vi "更新update.vi"() -> ()   [LabVIEW 2016, in "自动更新.lvlib"]
panel:
  out "waittime":u8
  out "下载的文件名":string
  out "更新进度":u8(slide) scale=0.0..100.0
  # "更新update，请稍后！"
  # "s"
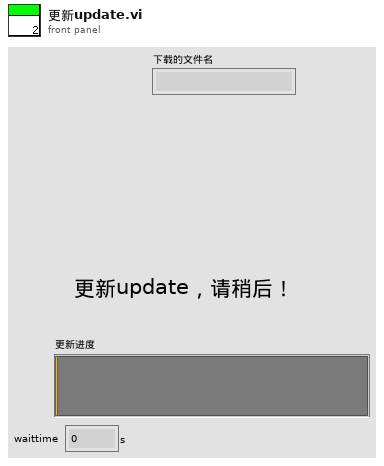
[diagram p1: front panel]
types:
  T1 = enum16{"get version information", "get success", "contact", "over"}
  T2 = cluster{"网络灯":bool, "接收中":bool, "已接收百分比":u8, "接收成功次数":dbl, "当前步骤":enum16{"init", "receivehead", "receivecontent", "receivesuccess", "over"}, "文件名":string, "error out":errorcluster}
  T3 = enum32{"Bad", "Idle", "Run top level", "Running"}
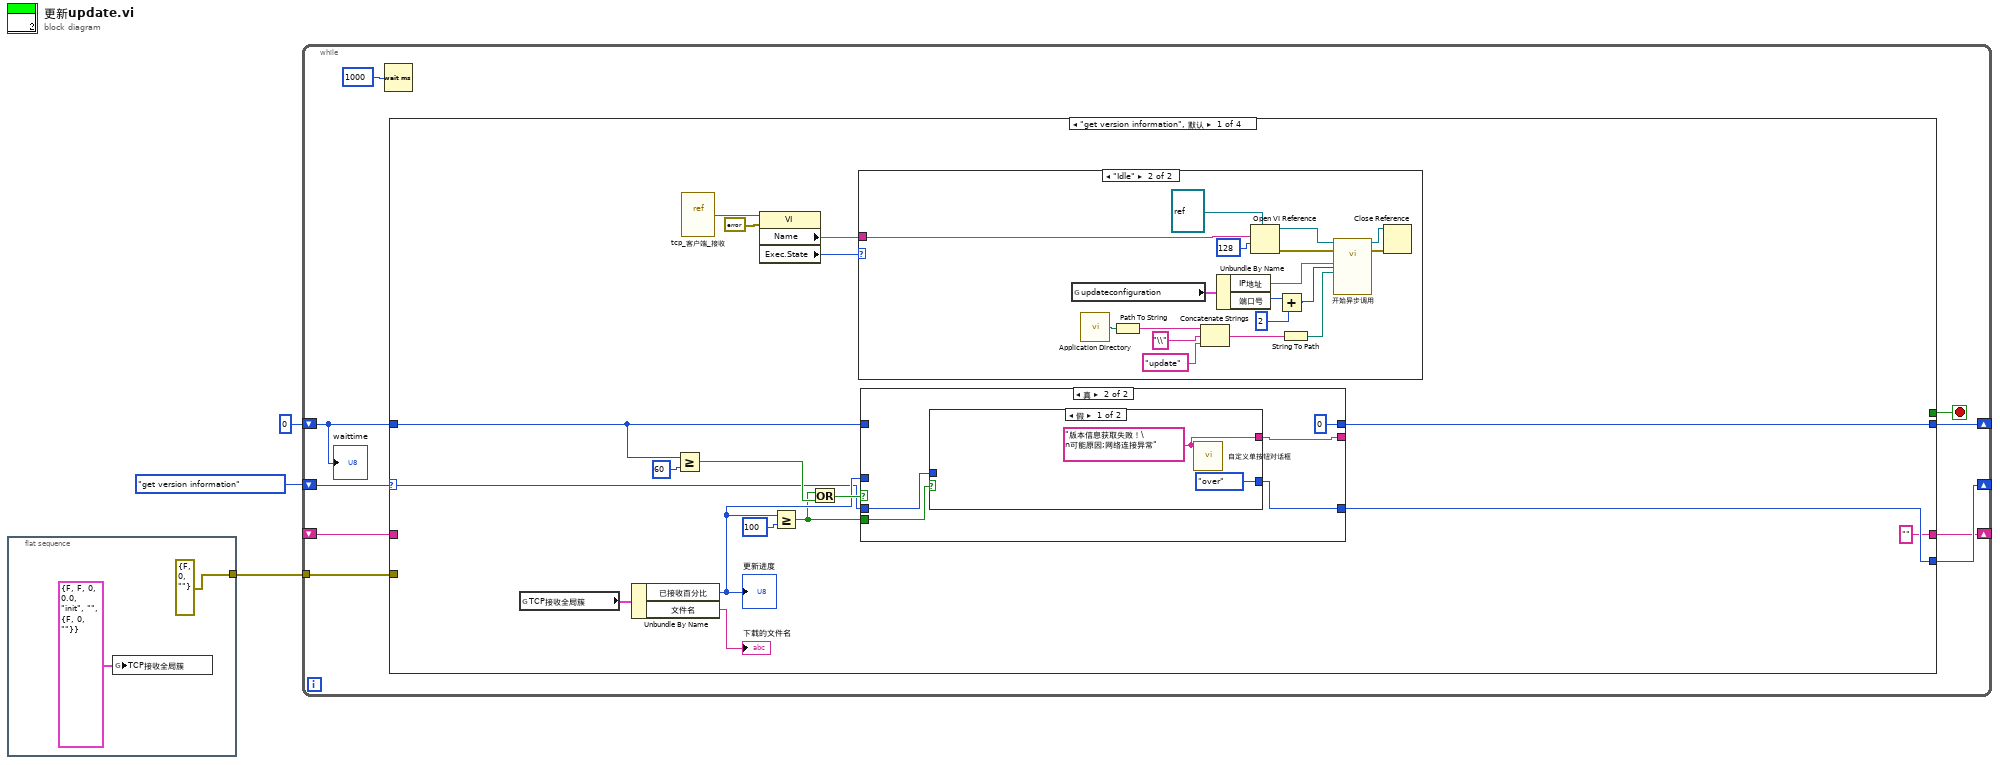
[diagram p0: block diagram]
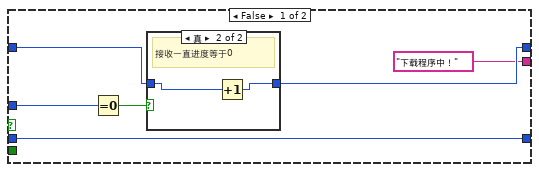
[diagram p2: hidden frame]
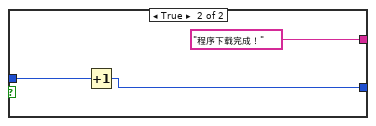
[diagram p4: hidden frame]
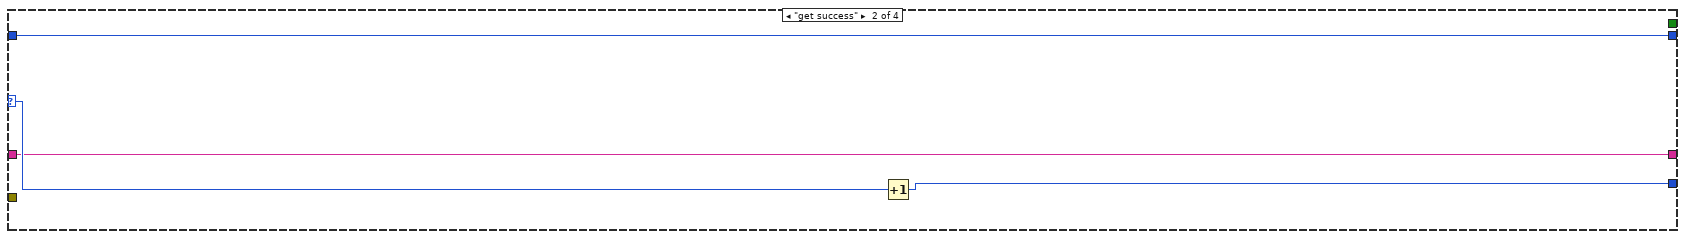
[diagram p6: hidden frame]
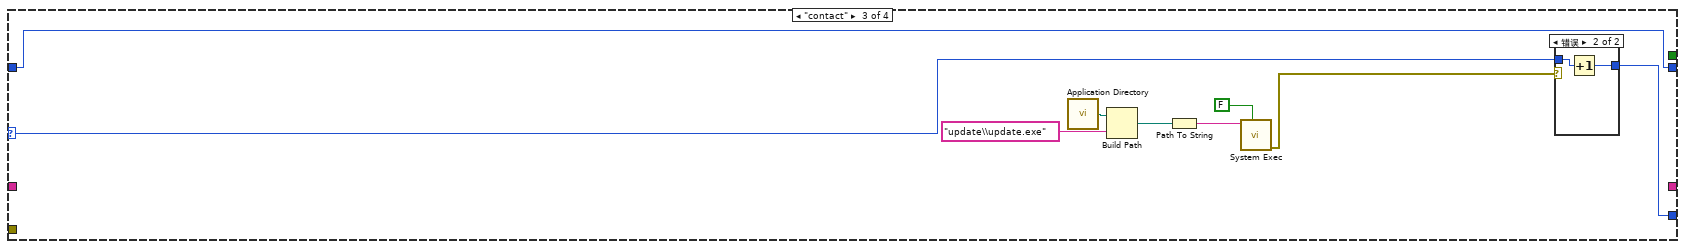
[diagram p7: hidden frame]
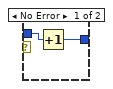
[diagram p8: hidden frame]
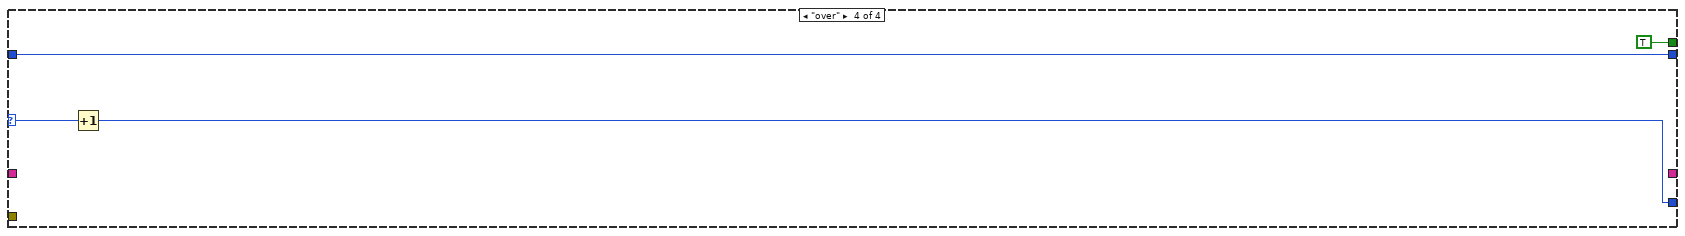
[diagram p9: hidden frame]
diagram:
  n1 = flat-sequence {
    tunnel: [errorcluster {"status"=FALSE, "code"=0, "source"=""} ("错误常量")] -> w1
    frame #0 {
      n2 = global write "全局变量1.vi" "TCP接收全局簇"(T2 {"网络灯"=FALSE, "接收中"=FALSE, "已接收百分比"=0, "接收成功次数"=0.0, "当前步骤"=enum."init", "文件名"="", "error out"={"status"=FALSE, "code"=0, "source"=""}} ("TCP接收全局簇")) -> ()
    }
  }
  n3 = while {
    shift-right: [w10] -> _
    shift-left: T1."get version information" -> [w13]
    shift-right: [w11] -> _
    shift-left: u8 0 ("y") -> [w12]
    tunnel: w1 -> [w9]
    shift-right: [w8] -> _
    shift-left: _ -> [w7]
    stop <- w6 stop-if-true
    n4 = Wait (ms)(milliseconds to wait=u32 1000 ("等待时间（毫秒）")) -> ()  [unwired: 1 out]
    n5 = case shown="\"get version information\", 默认" w13 {
      selector: w13 -> [w17 w71 w74 w87]
      tunnel: w12 -> [w19 w72 w80 w88]
      tunnel: [w18 w72 w80 w88] -> w11
      tunnel: [w16 w70 w81 w86] -> w10
      tunnel: w9 -> [_ _ _ _]
      tunnel: ["" w69 _ _] -> w8
      tunnel: w7 -> [_ w69 _ _]
      tunnel: [_ _ _ TRUE] -> w6
      frame "get version information", Default {
        n6 = global read "全局变量1.vi" "TCP接收全局簇"() -> (w22:T2)
        n7 = Unbundle By Name(w22) -> ("已接收百分比"=w23:u8, "文件名"=→"下载的文件名":string)
        "更新进度" <- w23
        n8 = Greater Or Equal?(x=w19, y=u8 60) -> (x >= y?=w25:bool)
        n9 = vi-ref "tcp_客户端_接收.vi"() -> (w31:refnum<vi>)
        n10 = property class="VI"(reference=w31, error in=errorcluster {"status"=FALSE, "code"=0, "source"=""} ("错误输出")) -> ("Name"=w30:string, "Exec.State"=w28:T3)  [unwired: 2 out]
        n11 = Greater Or Equal?(x=w23, y=u8 100) -> (x >= y?=w21:bool)
        n12 = Or(x=w21, y=w25) -> (x .or. y?=w24:bool)
        n13 = case shown="\"Idle\"" w28 {
          tunnel: w30 -> [_ w68]
          frame "Bad", Default {
          }
          frame "Idle" {
            n14 = global read "update全局.vi" "updateconfiguration"() -> (w61:cluster{"IP地址":string, "端口号":i32})
            n15 = call <vilib>:"Application Directory.vi"() -> ("Application Directory"=w58:path)
            n16 = Path To String(path=w58) -> (string=w55:string)
            n17 = Concatenate Strings(w55, "\\" ("字符串"), "update" ("字符串")) -> (w59:string)
            n18 = Unbundle By Name(w61) -> ("IP地址"=w60:string, "端口号"=w53:i32)
            n19 = Open VI Reference(type specifier VI Refnum (for type only)=refnum<vi> refnum, vi path=w68, options=128 ("选项")) -> (vi reference=w66:refnum<vi>, error out=w64:errorcluster)  [unwired: 3 in]
            n20 = Add(x=w53, y=2) -> (x+y=w51:i32)
            n21 = String To Path(string=w59) -> (path=w54:path)
            n22 = call-by-ref "开始异步调用"(reference=w66, error in=w64, "IP地址"=w60, "端口号"=w51, "储存路径"=w54) -> (reference out=w62:refnum<vi>, error out=w63:errorcluster)  [unwired: 17 in]
            n23 = Close Reference(reference=w62, error in (no error)=w63) -> ()  [unwired: 1 out]
          }
        }
        n24 = case shown="真" w24 {
          tunnel: w19 -> [w37 _]
          tunnel: [w36 u8 0] -> w18
          tunnel: w23 -> [w34 _]
          tunnel: [w33 w41] -> w16
          tunnel: w17 -> [w33 w42]
          tunnel: ["下载程序中！" w43] -> _
          tunnel: w21 -> [_ w44]
          frame False {
            n25 = Equal To 0?(x=w34) -> (x = 0?=w35:bool)
            n26 = case shown="真" w35 {
              tunnel: w37 -> [w38 w40]
              tunnel: [w38 w39] -> w36
              frame False {
              }
              frame True {
                # "接收一直进度等于0"
                n27 = Increment(x=w40) -> (x+1=w39:u8)
              }
            }
          }
          frame True {
            n28 = case shown="假" w44 {
              tunnel: [w47 "程序下载完成！"] -> w43
              tunnel: w42 -> [_ w49]
              tunnel: [T1."over" w48] -> w41
              frame False {
                w47 = "版本信息获取失败！\n可能原因;网络连接异常"
                n29 = call "自定义单按钮对话框.vi"("消息"=w47) -> ()  [unwired: 11 in]
              }
              frame True {
                n30 = Increment(x=w49) -> (x+1=w48:T1)
              }
            }
          }
        }
      }
      frame "get success" {
        n31 = Increment(x=w71) -> (x+1=w70:T1)
      }
      frame "contact" {
        n32 = call <vilib>:"Application Directory.vi"() -> ("Application Directory"=w77:path)
        n33 = Build Path(base path=w77, name or relative path="update\\update.exe" ("字符串")) -> (appended path=w78:path)
        n34 = Path To String(path=w78) -> (string=w75:string)
        n35 = call <vilib>:"System Exec.vi"("wait until completion? (T)"=FALSE, "command line"=w75) -> ("error out"=w73:errorcluster)  [unwired: 6 in, 3 out]
        n36 = case shown="错误" w73 {
          tunnel: w74 -> [w83 w85]
          tunnel: [w82 w84] -> w81
          frame No Error {
            n37 = Increment(x=w83) -> (x+1=w82:T1)
          }
          frame Error {
            n38 = Increment(x=w85) -> (x+1=w84:T1)
          }
        }
      }
      frame "over" {
        n39 = Increment(x=w87) -> (x+1=w86:T1)
      }
    }
    "waittime" <- w12
  }
